vi "Read Profile Array.vi"(0 "Device ID (0)":i32, 5 "Read Req":T3 {"Profile Pos" items=["CURRENT", "OLDEST", "SPECIFY"]}, 9 "Data Size (0: Auto Size)":u32, 11 "error in (no error)":errorcluster {"code" format="%.0x"}) -> (3 "Profile Info":T1, 4 "Device ID out":i32, 6 "Header Array":u32[][](array[numeric]), 8 "Height Profile Array":dbl[][](array[numeric]), 10 "Luminance Profile Array":u16[][](array[numeric]), 14 "Profile Rsp":T2, 15 "error out":errorcluster {"code" format="%.0x"})   [LabVIEW 2020, in "KEYENCE LJ-X8000A.lvlib"]
doc: "This function gets profile data.\nThe height and brightness profile data are each stored in a simple array.\nThe height profile is in units of mm."
uses:
  KEYENCE LJ-X8000A.lvlib
  Clusters/Read Profile Req.ctl
  Constants/Profile Pos.ctl
  Clusters/Read Profile Rsp.ctl
  Clusters/Profile Info.ctl
panel:
  # "(c) 2019 KEYENCE CORPORATION.  ALL RIGHTS RESERVED."
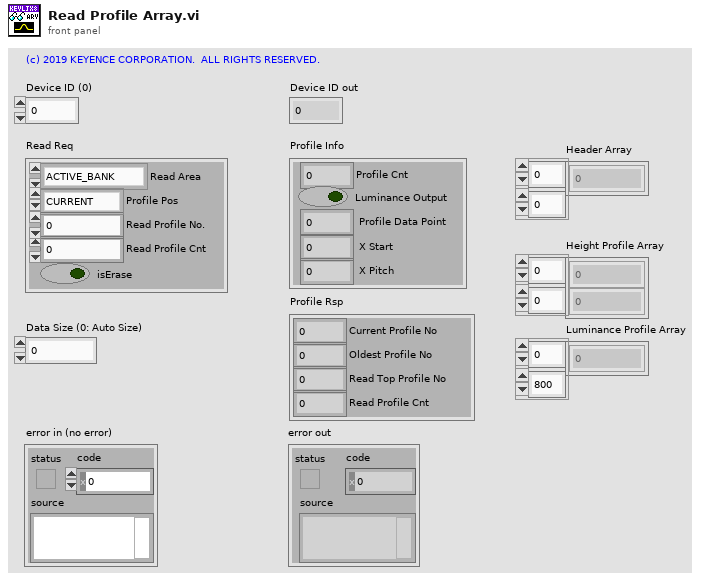
[diagram p1: front panel]
types:
  T1 = typedef "KEYENCE LJ-X8000A.lvlib/Profile Info.ctl" = cluster{"Profile Cnt":u8, "Luminance Output":bool, " Profile Data Point":u16, " X Start":i32, " X Pitch":i32}
  T2 = typedef "KEYENCE LJ-X8000A.lvlib/Read Profile Rsp.ctl" = cluster{"Current Profile No":u32, "Oldest Profile No":u32, "Read Top Profile No":u32, "Read Profile Cnt":u8}
  T3 = typedef "KEYENCE LJ-X8000A.lvlib/Read Profile Req.ctl" = cluster{"Read Area":enum8{"ACTIVE_BANK", "INACTIVE_BANK"}, "Profile Pos":T4, "Read Profile No.":u32, "Read Profile Cnt":u8, "isErase":bool}
  T4 = typedef "KEYENCE LJ-X8000A.lvlib/Profile Pos.ctl" = u8
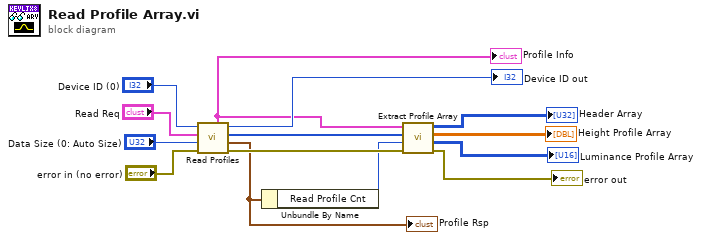
[diagram p0: block diagram]
diagram:
  n1 = call "Read Profiles.vi"("error in (no error)"="error in (no error)", "Data Size (0: Auto Size)"="Data Size (0: Auto Size)", "Read Req"="Read Req", "Device ID (0)"="Device ID (0)") -> ("error out"=w4:errorcluster, "Profile Rsp"=w2:T2, "Profile Data"=w9:u32[], "Device ID out"=→"Device ID out":i32, "Profile Info"=w8:T1)  [unwired: 3 in]
  "Profile Rsp" <- w2
  "Profile Info" <- w8
  n2 = Unbundle By Name(w2) -> ("Read Profile Cnt"=w1:u8)
  n3 = call "Extract Profile Array.vi"("error in (no error)"=w4, "Profile Cnt"=w1, "Profile Data"=w9, "Profile Info"=w8) -> ("error out"=→"error out":errorcluster, "Luminance Profile Array"=→"Luminance Profile Array":u16[][], "Height Profile Array"=→"Height Profile Array":dbl[][], "Header Array"=→"Header Array":u32[][])  [unwired: 4 in]
